vi "Preview.vi"(8 "error in (no error)":errorcluster, 11 "BroadcastRegistry in":refnum<class "BroadcastRegistry.lvclass">) -> (0 "error out":errorcluster, 2 "Registry":variant, 3 "BroadcastRegistry out":refnum<class "BroadcastRegistry.lvclass">)   [LabVIEW 2020, in "Communicable State Machine.lvlib" / "BroadcastRegistry.lvclass"]
uses:
  BroadcastRegistry.lvclass
  BroadcastRegistry.lvclass/BroadcastRegistry.ctl
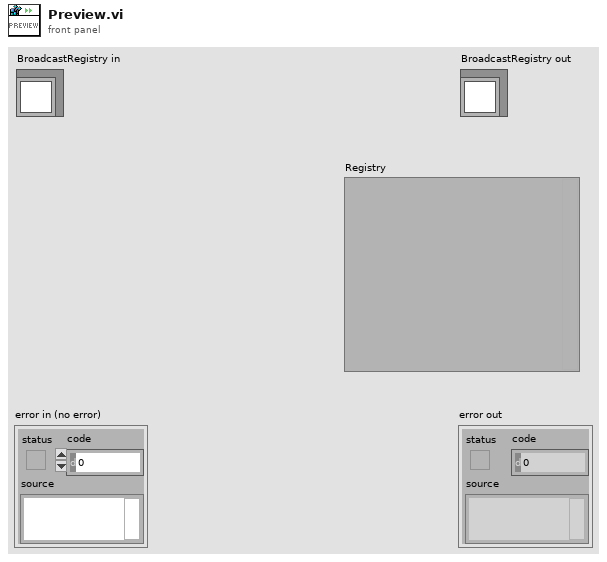
[diagram p1: front panel]
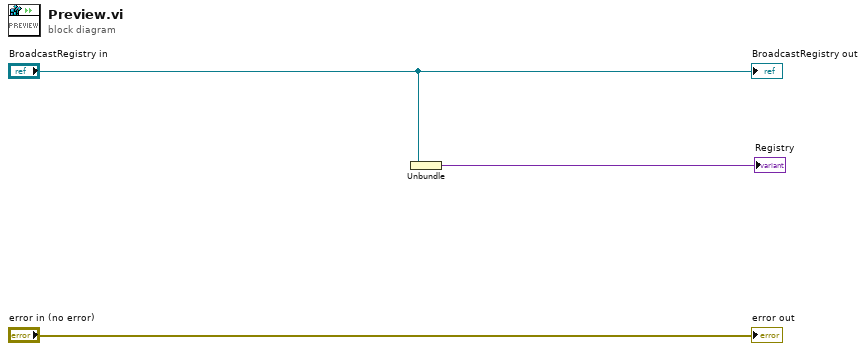
[diagram p0: block diagram]
diagram:
  n1 = Unbundle("BroadcastRegistry in") -> (→"Registry":variant)
  "error out" <- "error in (no error)"
  "BroadcastRegistry out" <- "BroadcastRegistry in"
